vi "Destroy Sync Context.vi"(8 "error in (no error)":errorcluster, 11 "SyncManager in":refnum<class "SyncProvider.lvclass">) -> (0 "error out":errorcluster, 3 "SyncManager out":refnum<class "SyncProvider.lvclass">)   [LabVIEW 2020, in "Instrument.lvlib" / "SyncProvider.lvclass"]
uses:
  SyncProvider.lvclass
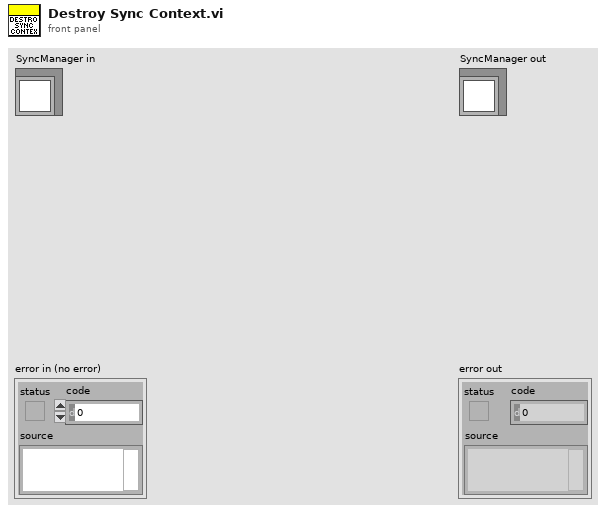
[diagram p1: front panel]
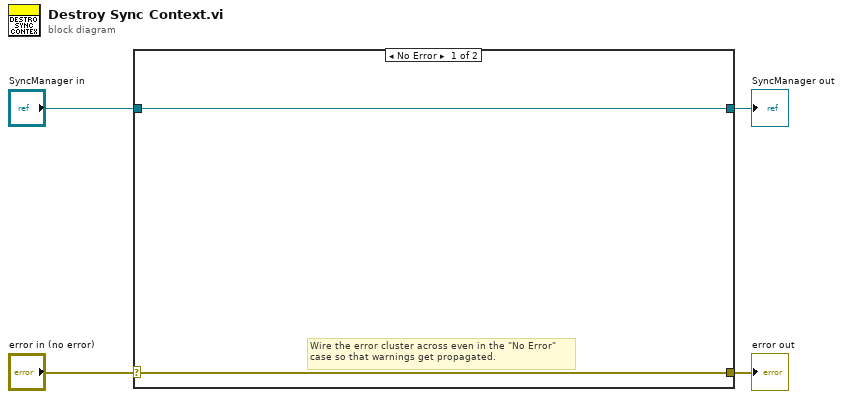
[diagram p0: block diagram]
diagram:
  n1 = case shown="No Error" "error in (no error)" {
    selector: "error in (no error)" -> [w5 w8]
    tunnel: [w5 w8] -> w3
    tunnel: [w6 w7] -> w1
    tunnel: "SyncManager in" -> [w6 w7]
    frame No Error {
      # "Wire the error cluster across even in the \"No Error\"\ncase so that warnings get propagated."
    }
    frame Error {
    }
  }
  "error out" <- w3
  "SyncManager out" <- w1
